vi "prototype UI_RESONANT.vi"() -> ()   [LabVIEW 2012]
uses:
  Custom Controls/Ch selector.ctl
  Custom Controls/MAIN Image panel reso tab Control type def.ctl
  Custom Controls/scan mode main settings tab.ctl
  Custom Controls/pixel resolution enum.ctl
  Custom Controls/advanced settings inner tab CTL.ctl
  Custom Controls/Histogram tab reso.ctl
  Custom Controls/file format type def.ctl
  Custom Controls/experiment type.ctl
  Custom Controls/display palette control.ctl
  <vilib>/event_ctls.llb/lveventtype.ctl
  GFG/GFG library.lvlib
panel:
  in  "reset zoom":bool
  in  "bool.stage.speed":bool
  in  "Objective":u16(ring) items=["10x Olympus", "20x Nikon", "30x Zeiss"]
  in  "x.voltage":dbl=0.9999999999999999 min=0.0 max=5.5 step=0.1
  in  "y.voltage":dbl=1.0 min=0.0 max=5.5 step=0.1
  in  "y.volt.offset":dbl=-0.2 step=0.1
  in  "x.volt.offset":dbl=-0.2 step=0.1
  in  "shutter":bool
  in  "x.pixels":i32=256 min=2 max=2048 step=2
  in  "clear prot":bool
  in  "timestamp.prot":bool
  in  "protocol.notes":string caption="notebook"
  in  "pos \nstore F":bool
  in  "pos \nstore E":bool
  in  "pos \nstore D":bool
  in  "pos \nstore C":bool
  in  "pos \nstore B":bool
  in  "pos \nstore A":bool
  out "String 10":string
  in  "pos \nrecall F":bool
  in  "pos \nrecall E":bool
  in  "pos \nrecall D":bool
  in  "pos \nrecall C":bool
  in  "pos \nrecall B":bool
  in  "pos \nrecall A":bool
  out "String 11":string
  in  "ref img\nOpen Files Button":bool
  in  "ref img\nstore F":bool
  in  "ref img\nstore E":bool
  in  "ref img\nstore D":bool
  in  "ref img\nstore C":bool
  in  "ref img\nstore B":bool
  in  "ref img\nstore A":bool
  out "String 17":string
  in  "ref img\nSave As Button":bool
  in  "Open All\nSettings":bool
  in  "step.size.z":u16(ring)=6 items=["  1"=1, "  2"=2, "  5"=5, " 10"=10, " 20"=20, " 50"=50, "100"=100]
  in  "Stage Stop":bool
  out "frame count":dbl(slide) scale=-1.0..500.0
  in  "scan mode main settings":T1
  in  "x.correction":dbl(slide)=30.0 min=-100.0 max=100.0 step=1.0 scale=-100.0..100.0 scale format="%#_3g"
  in  "Start.Delay":dbl(slide)=220.0 min=1.0 max=320.0 step=1.0 scale=1.0..320.0 scale format="%#_3g"
  in  "pixel resolution":T2
  in  "ZOOM":dbl(slide)=1.0 min=1.0 max=16.0 step=0.1 scale=1.0..16.0 scale format="%_2g"
  in  "no. of frames to acquire":i32=10000 min=2 max=2147483646 step=2
  in  "x.fov":dbl caption="Field of view    x" format="%#_3p"
  in  "y.fov":dbl caption="y" format="%#_3p"
  out "frames.p.sec":dbl caption="frames/s" format="%#.2g"
  in  "resonant.correction.enable":bool
  out "pixels per line":i32=10000 min=2 max=2147483646 step=2
  out "lines per second":i32=10000 min=2 max=2147483646 step=2
  in  "linescan.y.pixels":i32=256 caption="Lines to display at once" min=2 max=2048 step=2
  in  "no. of lines to acquire":i32=10000 min=2 max=2147483646 step=2
  in  "save.ch.1":bool caption="ch 1"
  in  "save.ch.2":bool caption="ch 2"
  in  "save.ch.3":bool caption="ch 3"
  in  "save.ch.4":bool caption="ch 4"
  in  "save.ch.5":bool caption="ch 5"
  in  "experiment type":T3
  in  "experiment name":string
  in  "root.path":path=path "g:/"
  in  "file format":T4
  out "stack.duration":i32=10 caption="stack.duration (sec)" min=0 max=2147483646 step=2
  in  "add":bool
  in  "clear all":bool
  in  "clear last":bool
  in  "move to z.stack.\nstart plane":bool
  in  "start z.stack":bool
  in  "frames.per.plane":i32=10000
  in  "z.spacing":dbl=1.0 caption="z.spacing (um)" min=0.1 step=0.1
  out "no of planes":i32=10 min=0 max=2147483646 step=2
  in  "piezo.mode":bool
  in  "frames.per.z.cycle":dbl=2.0 min=3.0 max=101.0 step=2.0
  in  "piezo.active":bool
  in  "Z UP":bool
  in  "Z DOWN":bool
  out "String 7":string
  in  "step.size.xy":u16(ring)=6 items=["  1"=1, "  2"=2, "  5"=5, " 10"=10, " 20"=20, " 50"=50, "100"=100]
  in  "Y UP":bool
  in  "X LEFT":bool
  in  "Y DOWN":bool
  in  "X RIGHT":bool
  out "String 6":string
  in  "setY":dbl caption="Z-Stepper" format="%#.1f"
  in  "setX":dbl caption="Z-Stepper" format="%#.1f"
  in  "setZ":dbl caption="set" format="%#.1f"
  out "String 4":string
  out "posZ":dbl caption="actual" format="%#.1f"
  out "posX":dbl caption="Z-Stepper" format="%#.1f"
  out "posY":dbl caption="Z-Stepper" format="%#.1f"
  out "String 3":string
  in  "QUIT":bool
  in  "Record":bool
  in  "FOCUS":bool
  in  "MAIN Image panels reso":T5
  out "Channel 1 large":T6(plugin-control)
  out "Channel 2 large":T6(plugin-control)
  out "Channel 3 large":T6(plugin-control)
  out "Channel 4 large":T6(plugin-control)
  out "Channel 5 large":T6(plugin-control)
  out "Channel 1 small":T6(plugin-control)
  out "Channel 2 small":T6(plugin-control)
  out "Channel 4 small":T6(plugin-control)
  out "Channel 3 small":T6(plugin-control)
  in  "Blue Channel (Overlay)":T7 caption="B"
  in  "Green Channel (Overlay)":T7=enum."Ch 1" caption="G"
  in  "Red Channel (Overlay)":T7=enum."Ch 2" caption="R"
  out "RGB overlay":T6(plugin-control)
  out "ROI chart":sgl[][](graph)=[[54.570076, 54.556858]]
  in  "ROI channel":T7=enum."Ch 1" caption="Channel"
  out "ROI Image display":T6(plugin-control)
  in  "confirm line":bool
  in  "channel arb line scan":T7 caption="Channel"
  out "arb line scan display":T6(plugin-control)
  in  "Cancel":bool
  in  "hist/ref slider tab":enum32{" "}(tab)
  in  "display every n-th frame":i8=4 min=2 step=1
  in  "PIN Button hist/ref slider tab":bool
  in  "Histograms tab reso":T8
  in  "auto scale\n      CH 1":bool=TRUE caption="auto scale 2"
  in  "Min Max Channel 1":cluster{dbl, dbl}(slide) scale=-32768.0..32767.0 scale format="%#_5g"
  out "Histogram 1":T9(graph)
  out "String 12":string
  in  "auto scale\n      CH 4":bool=TRUE caption="auto scale 2"
  in  "Min Max Channel 4":cluster{dbl, dbl}(slide) scale=-100.0..2047.0 scale format="%#_4g"
  out "Histogram 4":T9(graph)
  out "String 15":string
  in  "auto scale\n      CH 5":bool=TRUE caption="auto scale 2"
  in  "Min Max Channel 5":cluster{dbl, dbl}(slide) scale=-100.0..2047.0 scale format="%#_4g"
  out "Histogram 5":T9(graph)
  out "String 16":string
  in  "auto scale\n      CH 3":bool=TRUE caption="auto scale 2"
  in  "Min Max Channel 3":cluster{dbl, dbl}(slide) scale=-32768.0..32767.0 scale format="%#.1f"
  out "Histogram 3":T9(graph)
  out "String 14":string
  in  "auto scale\n      CH 2":bool=TRUE caption="auto scale 2"
  in  "Min Max Channel 2":cluster{dbl, dbl}(slide) scale=-32768.0..32767.0 scale format="%#.0f"
  out "Histogram 2":T9(graph)
  out "String 13":string
  in  "avg type":u16(ring) items=["none", "group avg", "moving avg"]
  in  "avg of":i8=10 min=2 step=1
  in  "display palette":T10
  in  "laser power slider tab":enum32{""}(tab)
  in  "enable set power max":bool
  in  "set power max":bool
  in  "Laser Power":dbl(knob) min=0.0 max=100.0 step=0.5 scale=0.0..100.0 scale format="%3d"
  in  "PIN Button laser power slider tab":bool
  in  "PMT slider tab":enum32{""}(tab)
  in  "PMT 2":u16(slide) max=1000 scale=0.0..1000.0
  in  "PMT 1":u16(slide) max=1250 scale=0.0..1000.0
  out "String 5":string
  in  "PMT 4":u16(slide) max=1000 scale=0.0..1000.0
  in  "PMT 3":u16(slide) max=1250 scale=0.0..1000.0
  out "String 18":string
  in  "PIN Button PMT slider tab":bool
  in  "advanced settings slider tab":enum32{""}(tab)
  in  "advanced settings inner tab":T11
  in  "y.pixel.sz":dbl=1e-05 min=1e-09 max=1e-05 step=1e-07 format="%#_3p"
  in  "x.pixel.sz":dbl=1e-05 min=1e-09 max=1e-05 step=1e-07 format="%#_3p"
  in  "y.pixels":i32=256 caption="Y Resolution" min=2 max=2048 step=2
  in  "nomin.x.pixels":i32=256 caption="X resolution" min=2 max=2048 step=2
  in  "voltage.for\nmin.field.of.view\nresonant":dbl=5.0
  in  "max.field.of.view\nresonant":dbl=300.0 format="%#_6p"
  in  "voltage.for\nmax.field.of.view\nresonant":dbl=5.0
  in  "max.field.of.view":dbl=300.0 format="%#_6p"
  in  "voltage.for\nmax.field.of.view":dbl=5.0
  in  "external.start.trigger.enable":bool=TRUE caption="WAIT FOR TRIGGER"
  in  "pos  pockels cell PMT Data":dbl[][](array[numeric])=[[0.0, 0.0], [1.0, 0.0]] caption="Data" format="%0.1f"
  out "interpol XY":cluster{dbl[], "Best Exponential Fit":dbl[]}[](graph)
  in  "PIN Button advanced settings slider tab":bool
  in  "XYZ stage settings slider tab":enum32{" "}(tab)
  in  "set stage speed":bool
  in  "enable virtual XYZ":bool
  out "String 19":string
  in  "set Y to zero":bool
  in  "set X to zero":bool
  in  "set all to zero":bool
  in  "set Z to zero":bool
  out "String 9":string
  in  "reverse y":bool
  in  "reverse x":bool
  in  "reverse z":bool
  out "String 8":string
  in  "PIN Button XYZ stage settings slider tab":bool
  in  "SCIENTIFICA Button":bool
  # "to zoom out press and hold Shift"
  # "current pos."
  # "go to pos."
  # "STORE positions"
  # "RECALL  positions"
  # "REFERENCE IMAGES"
  # "STORE"
  # "CHANNELS TO SAVE"
  # "zig-zag (leaf scan)"
  # "planes"
  # "1"
  # "2"
  # "3"
  # "4"
  # "Press and hold Ctrl to add multiple ROIs"
  # "This checkbox is only for starting the image acquisition using a TTL rising edge trigger from an external device. Don't tick this box unless an incoming trigger is wired up, otherwise the software may freeze. To reset, click QUIT and restart. If you want to send a trigger to an external device, just connect the ai.start.trigger.channel (e.g.PFI2, specified in settings.INI) to the external device, but leave the  checkbox above unticked."
  # "Z"
  # "laser"
  # "virtual XYZ"
  # "set zero"
  # "reverse \ndirection"
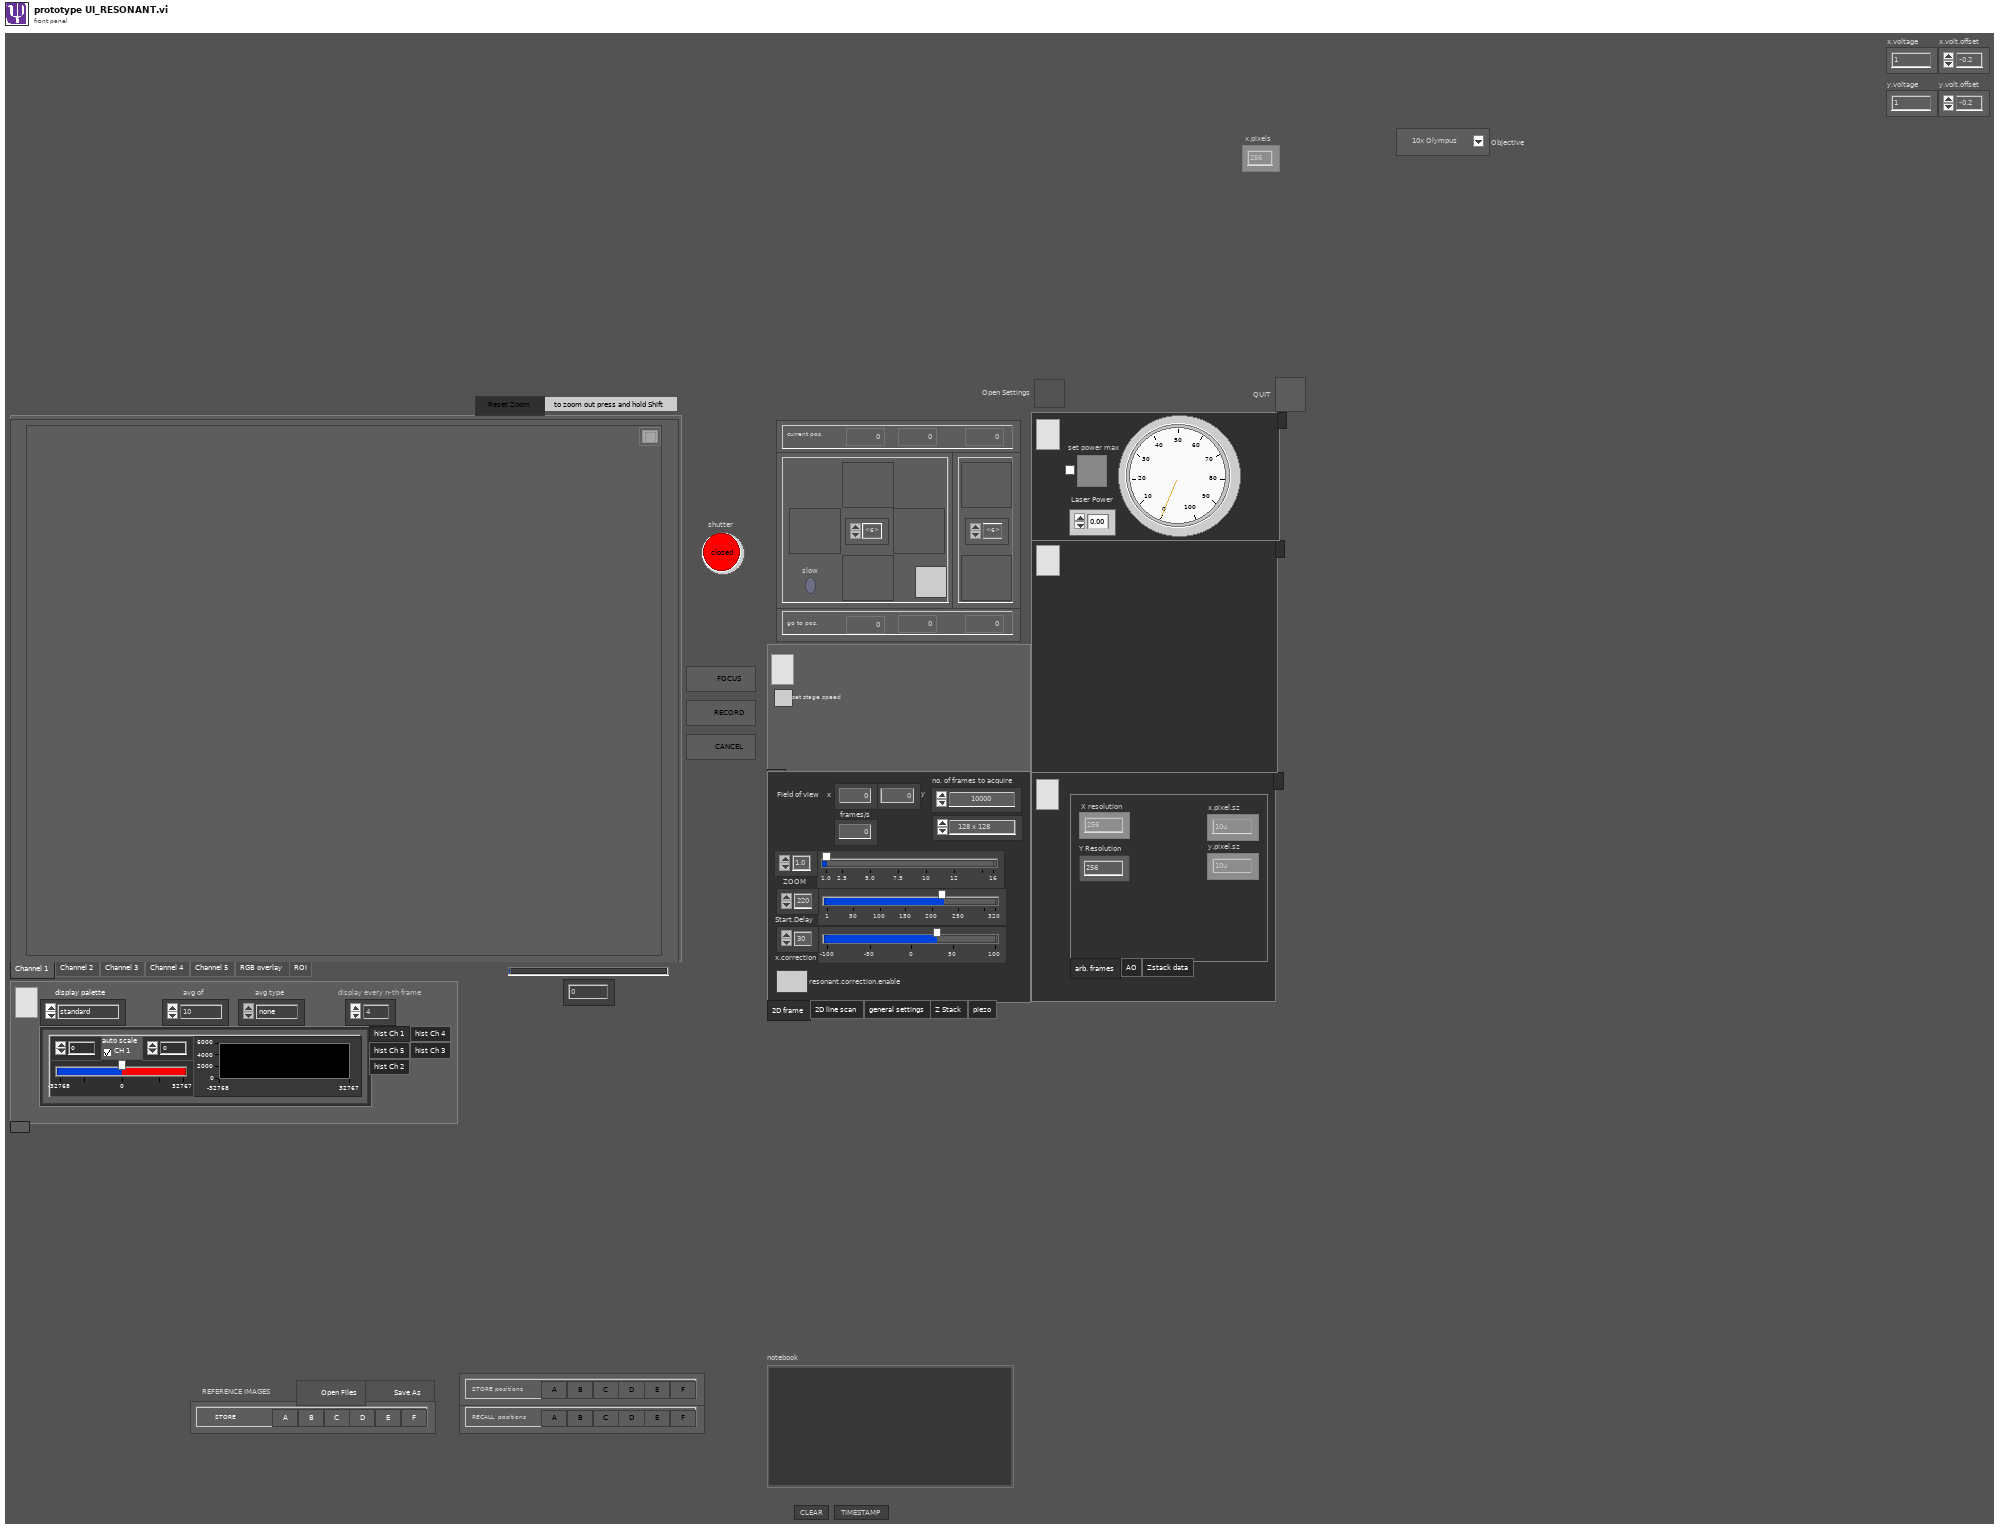
[diagram p1: front panel]
types:
  T1 = typedef "scan mode main settings tab.ctl" = enum32{"2D frame", "2D line scan", "general settings", "Z Stack", "piezo"}
  T2 = typedef "pixel resolution enum.ctl" = enum16{"   128 x 128", "   256 x 128", "   256 x 256", "   512 x  64", "   512 x 128", "   512 x 256", "   512 x 512", "  1024 x 512", "  1024 x 1024", "   arbitrary"}
  T3 = typedef "experiment type.ctl" = string
  T4 = typedef "file format type def.ctl" = enum16{"16bit raw", "32bit raw", "16bit multi-tiff (interleave)", "16bit multi-tiff (separate)", "16bit multi-tiff (stacked)", "32bit multi-tiff (interleave)", "32bit multi-tiff (separate)", "32bit multi-tiff (stacked)", "16bit tiff series (interleave)", "16bit tiff series (separate)", "16bit tiff series (stacked)", "32bit tiff series (interleave)", "32bit tiff series (separate)", "32bit tiff series (stacked)"}
  T5 = typedef "MAIN Image panel reso tab Control type def.ctl" = enum32{"Channel 1", "Channel 2", "Channel 3", "Channel 4", "Channel 5", "all channels", "RGB overlay", "ROI", "arbitrary line scan"}
  T6 = typedef "IMAQ Image.ctl" = refnum<image>
  T7 = typedef "Ch selector.ctl" = enum16{"none", "Ch 1", "Ch 2", "Ch 3", "Ch 4", "Ch 5"}
  T8 = typedef "Histogram tab reso.ctl" = enum32{"hist Ch 1", "hist Ch 4", "hist Ch 5", "hist Ch 3", "hist Ch 2"}
  T9 = cluster{"Starting Value":sgl, "Incremental Value":sgl, "Histogram":u32[]}
  T10 = typedef "display palette control.ctl" = enum16{"standard", "high clipping red", "low clipping blue", "high and low clipping"}
  T11 = typedef "advanced settings inner tab CTL.ctl" = enum32{"arb. frames", "AO", "AI", "channels", "trigger", "Zstack data"}
  T12 = enum8{"Enabled", "Disabled", "Disabled and Grayed Out"}
  T13 = typedef "Image Type" = u32
  T14 = cluster{refnum<vi>, refnum<vi>, refnum<vi>, refnum<vi>, refnum<vi>, refnum<vi>, refnum<vi>, refnum<vi>, refnum<vi>, refnum<vi>, refnum<vi>, refnum<vi>}
  T15 = cluster{"New Image":T6, "New Image":T6, "New Image":T6, "New Image":T6, "New Image":T6, "New Image":T6, "New Image":T6, "New Image":T6, "New Image":T6, "New Image":T6, "New Image":T6, "New Image":T6}
  T16 = typedef "lveventtype.ctl" = enum32{"Null", "Timeout", "Annotation Menu Selection", "Annotation Menu Selection?", "App Instance Close", "App Instance Close?", "Autoscale Range Change", "Cell Edit", "Cell Edit?", "Cursor Grab", "Cursor Grab?", "Cursor Menu Selection", "Cursor Menu Selection?", "Cursor Move", "Cursor Release", "Data Change", "Direction Change", "Display State Change", "Drag Ended", "Drag Enter", "Drag Leave", "Drag Over", "Drag Source Update", "Drag Starting", "Drag Starting?", "Drop", "Exec State Change", "Key Down", "Key Down?", "Key Repeat", "Key Repeat?", "Key Up", "Listbox Double Click", "Menu Activation?", "Menu Selection (App)", "Menu Selection? (App)", "Menu Selection (User)", "Mouse Down", "Mouse Down?", "Mouse Enter", "Mouse Leave", "Mouse Move", "Mouse Up", "NI Security User Change (App)", "Pane Size", "Panel Close", "Panel Close?", "Panel Resize", "Plot Attribute Change", "Scale Range Change", "Shortcut Menu Activation?", "Shortcut Menu Selection (App)", "Shortcut Menu Selection? (App)", "Shortcut Menu Selection (User)", "Tree Double Click", "Tree Drag", "Tree Drag?", "Tree Drop", "Tree Drop?", "Tree Item Close", "Tree Item Close?", "Tree Item Open", "Tree Item Open?", "Value Change"}
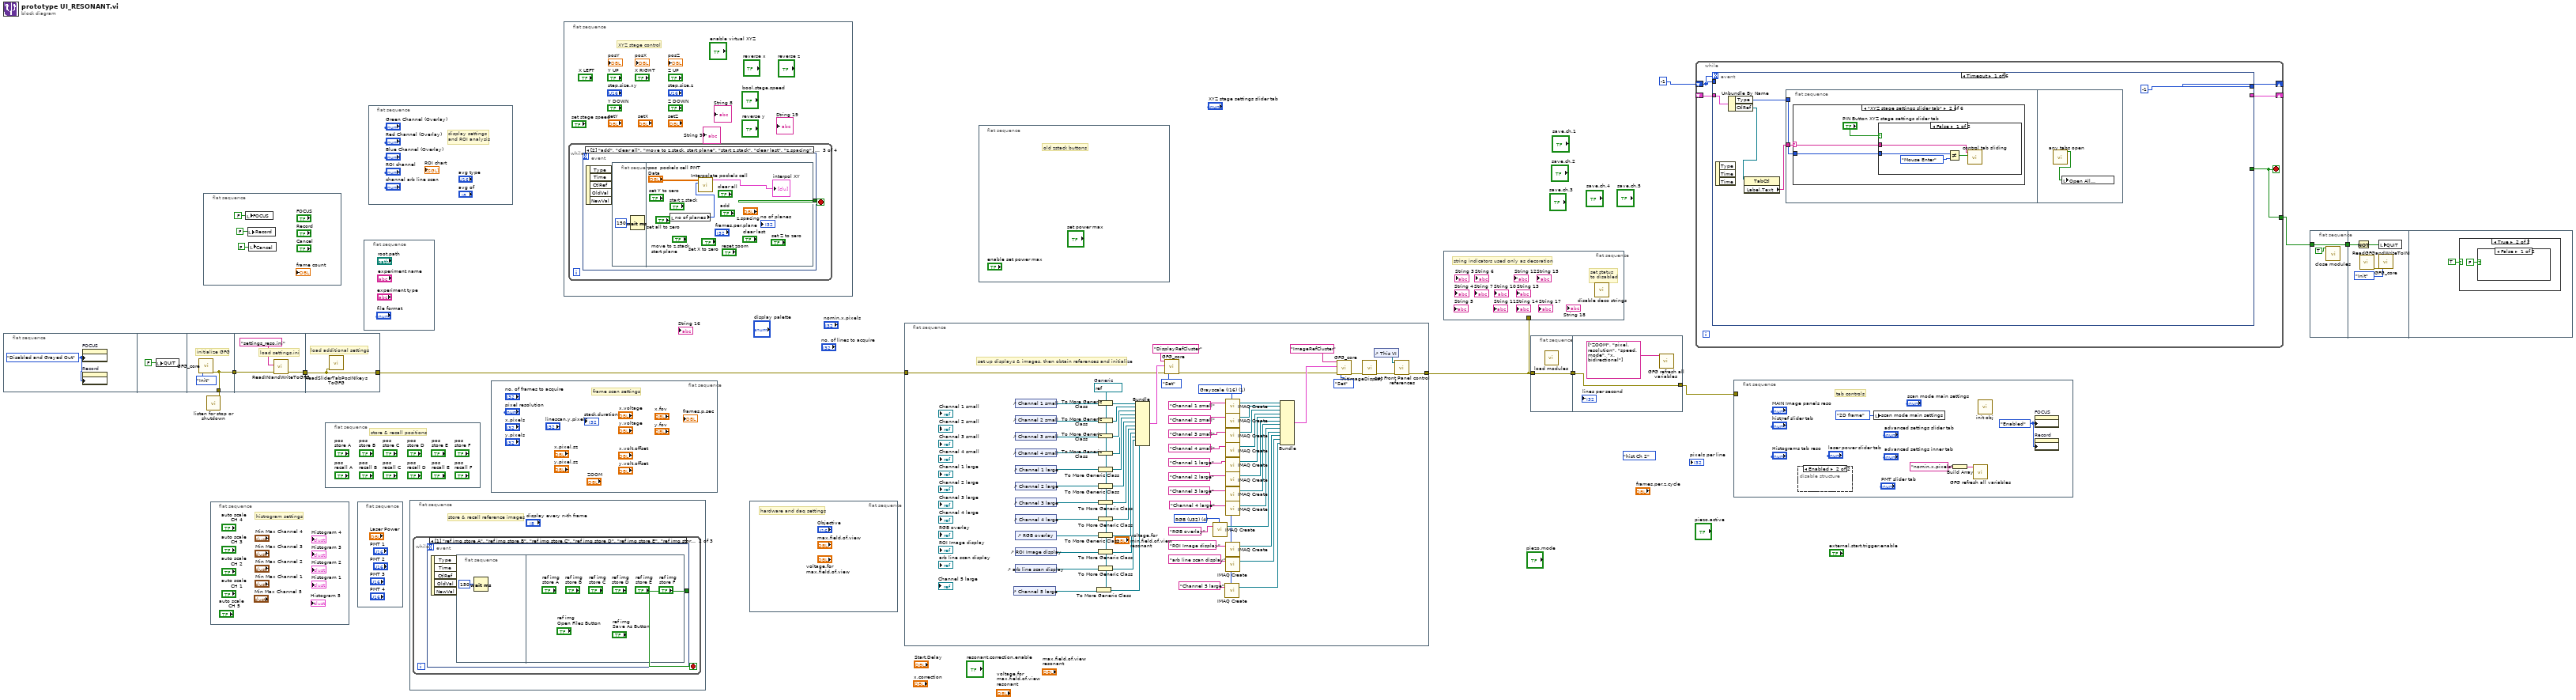
[diagram p0: block diagram]
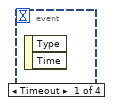
[diagram p2: hidden frame]
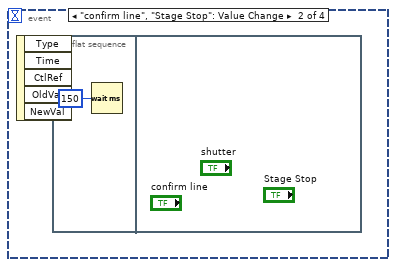
[diagram p3: hidden frame]
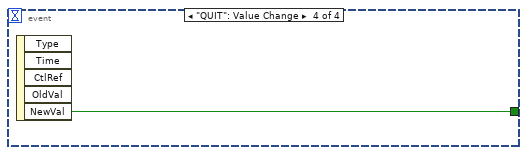
[diagram p4: hidden frame]
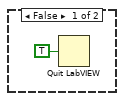
[diagram p5: hidden frame]
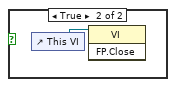
[diagram p6: hidden frame]
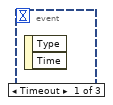
[diagram p7: hidden frame]
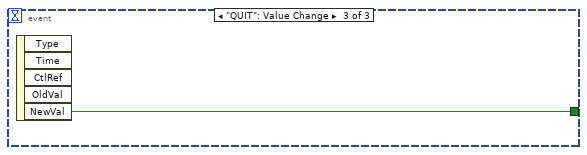
[diagram p8: hidden frame]
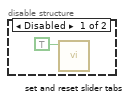
[diagram p9: hidden frame]
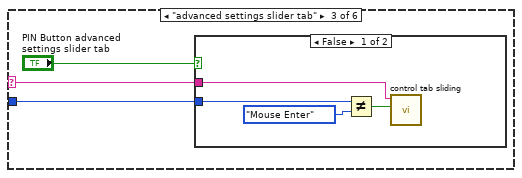
[diagram p12: hidden frame]
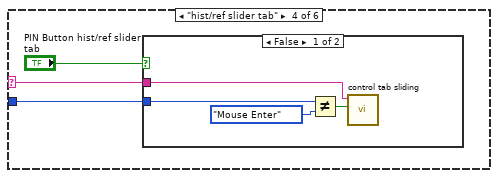
[diagram p14: hidden frame]
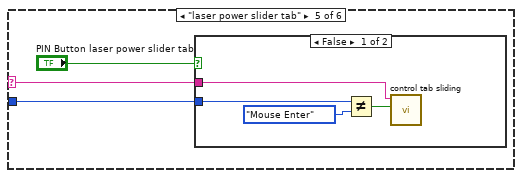
[diagram p16: hidden frame]
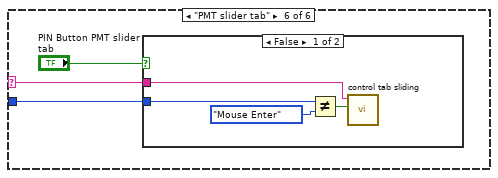
[diagram p18: hidden frame]
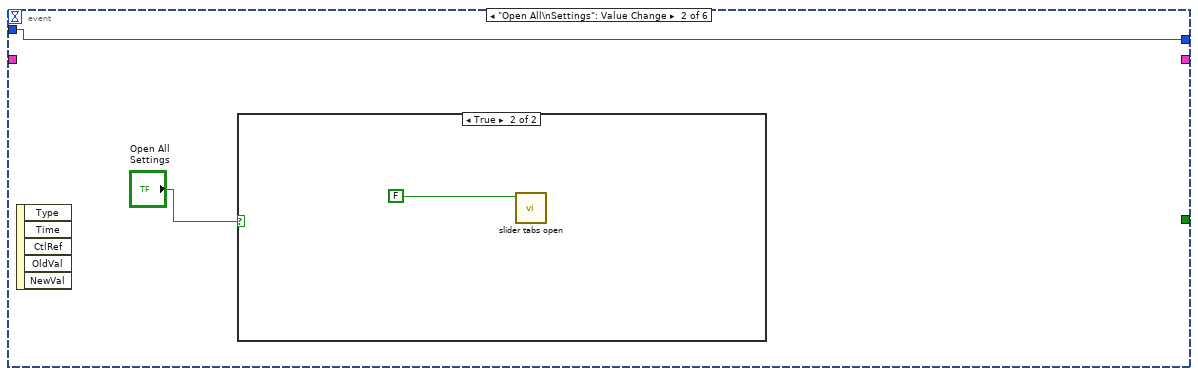
[diagram p20: hidden frame]
diagram:
  (unwired) Histogram_tab_reso."hist Ch 2" ("Histograms tab reso")
  n1 = flat-sequence {
    tunnel: [w13] -> w10
    tunnel: [w13] -> w9
    tunnel: w10 -> [w17]
    tunnel: [w16] -> w3
    tunnel: [w18] -> w6
    tunnel: w3 -> [w18]
    frame #0 {
      w11 = T12."Disabled and Grayed Out" ("Disabled")
      n2 = property on="FOCUS" class="Bool (strict)"("DisabledEnum"=w11) -> ()  [unwired: 2 in, 2 out]
      n3 = property on="Record" class="Bool (strict)"("DisabledEnum"=w11) -> ()  [unwired: 2 in, 2 out]
    }
    frame #1 {
      n4 = local write "QUIT"(FALSE ("QUIT")) -> ()
    }
    frame #2 {
      # "initialize GFG"
      n5 = call "GFG_core.vi"("Action"=enum16{"Init", "Set", "Get"}."Init") -> ("error out"=w13:errorcluster)  [unwired: 12 in, 6 out]
    }
    frame #3 {
      # "load settings.ini"
      n6 = call "ReadINIandWriteToGFG.vi"("error in (no error)"=w17, "name or relative path"="settings_reso.ini") -> ("error out"=w16:errorcluster)  [unwired: 9 in]
    }
    frame #4 {
      # "load additional settings"
      n7 = call "ReadSliderTabPosINIkeysToGFG.vi"("error in (no error)"=w18) -> ()  [unwired: 11 in]
    }
  }
  n8 = flat-sequence {
    frame #0 {
      n9 = local write "FOCUS"(FALSE ("FOCUS")) -> ()
      n10 = local write "Record"(FALSE ("Record")) -> ()
      n11 = local write "Cancel"(FALSE ("Cancel")) -> ()
    }
  }
  n12 = call "listen for stop or shutdown.vi"("error in (no error)"=w9) -> ()  [unwired: 9 in, 2 out]
  n13 = flat-sequence {
    frame #0 {
      # "histrogram settings"
    }
  }
  n14 = flat-sequence {
    frame #0 {
      # "store & recall positions"
    }
  }
  n15 = flat-sequence {
    frame #0 {
    }
  }
  n16 = flat-sequence {
    frame #0 {
    }
  }
  n17 = flat-sequence {
    frame #0 {
      # "display settings\nand ROI analysis"
    }
  }
  n18 = flat-sequence {
    frame #0 {
      # "store & recall reference images"
      n19 = while {
        stop <- w22 stop-if-true
        n20 = event shown="[1] \"ref img store A\", \"ref img store B\", \"ref img store C\", \"ref img store D\", \"ref img store E\", \"ref img store F\", \"ref img Save As Button\", \"ref img Open Files Button\": Value Change" {
          selector: _ -> [_ _ _]
          dyn-events: _ -> [_ _ _]
          timeout: _ -> [_ _ _]
          tunnel: [_ _ w24] -> w22
          event Timeout {
            n21 = event-data() -> ()  [unwired: 1 in, 2 out]
          }
          event "ref img\nstore A", "ref img\nstore B", "ref img\nstore C", "ref img\nstore D", "ref img\nstore E", "ref img\nstore F", "ref img\nSave As Button", "ref img\nOpen Files Button": Value Change {
            n22 = event-data() -> ()  [unwired: 1 in, 5 out]
            n23 = flat-sequence {
              frame #0 {
                n24 = Wait (ms)(milliseconds to wait=u32 150) -> ()  [unwired: 1 out]
              }
              frame #1 {
              }
            }
          }
          event "QUIT": Value Change {
            n25 = event-data() -> ("NewVal"=w24:bool)  [unwired: 1 in, 4 out]
          }
        }
      }
    }
  }
  n26 = flat-sequence {
    frame #0 {
      # "frame scan settings"
    }
  }
  n27 = flat-sequence {
    frame #0 {
      # "XYZ stage control"
      n28 = while {
        stop <- w25 stop-if-true
        n29 = event shown="[2] \"add\", \"clear all\", \"move to z.stack. start plane\", \"start z.stack\", \"clear last\", \"z.spacing\", \"frames.per.plane\", \"no of planes\", \"set Y to zero\", \"set X to zero\", \"set all to zero\", \"set Z to zero\", \"reset zoom\": Value Change" {
          selector: _ -> [_ _ _ _]
          dyn-events: _ -> [_ _ _ _]
          timeout: _ -> [_ _ _ _]
          tunnel: [_ _ _ w31] -> w25
          event Timeout {
            n30 = event-data() -> ()  [unwired: 1 in, 2 out]
          }
          event "confirm line", "Stage Stop": Value Change {
            n31 = event-data() -> ()  [unwired: 1 in, 5 out]
            n32 = flat-sequence {
              frame #0 {
                n33 = Wait (ms)(milliseconds to wait=u32 150) -> ()  [unwired: 1 out]
              }
              frame #1 {
              }
            }
          }
          event "add", "clear all", "move to z.stack.\nstart plane", "start z.stack", "clear last", "z.spacing", "frames.per.plane", "no of planes", "set Y to zero", "set X to zero", "set all to zero", "set Z to zero", "reset zoom": Value Change {
            n34 = event-data() -> ()  [unwired: 1 in, 5 out]
            n35 = flat-sequence {
              frame #0 {
                n36 = Wait (ms)(milliseconds to wait=u32 150) -> ()  [unwired: 1 out]
              }
              frame #1 {
                n37 = local read "no of planes"() -> (w30:i32)
                n38 = call "Interpolate pockels cell.vi"("nr of planes"=w30, "Data"="pos  pockels cell PMT Data") -> ("Raw Data and Interpolated Data"=→"interpol XY":cluster{dbl[], "Best Exponential Fit":dbl[]}[])  [unwired: 8 in, 1 out]
              }
            }
          }
          event "QUIT": Value Change {
            n39 = event-data() -> ("NewVal"=w31:bool)  [unwired: 1 in, 4 out]
          }
        }
      }
    }
  }
  n40 = flat-sequence {
    frame #0 {
      # "hardware and daq settings"
    }
  }
  n41 = flat-sequence {
    tunnel: [w51] -> w7
    tunnel: w6 -> [w50]
    frame #0 {
      w38 = T13 4 items=["Grayscale (U8)", "Grayscale (I16)", "Grayscale (SGL)", "Complex (CSG)", "RGB (U32)", "HSL (U32)", "RGB (U64)", "Grayscale (U16)"] ("Image Type")
      w33 = T13 1 items=["Grayscale (U8)", "Grayscale (I16)", "Grayscale (SGL)", "Complex (CSG)", "RGB (U32)", "HSL (U32)", "RGB (U64)", "Grayscale (U16)"] ("Image Type")
      w36 = refnum<vi> refnum  # Generic
      # "set up displays & images, then obtain references and initialize"
      n42 = control-ref of="Channel 5 large"() -> (w37:refnum<vi>)
      n43 = control-ref of="Channel 1 small"() -> (w49:refnum<vi>)
      n44 = control-ref of="Channel 2 small"() -> (w48:refnum<vi>)
      n45 = control-ref of="Channel 3 small"() -> (w47:refnum<vi>)
      n46 = control-ref of="Channel 4 small"() -> (w46:refnum<vi>)
      n47 = control-ref of="Channel 1 large"() -> (w45:refnum<vi>)
      n48 = control-ref of="Channel 2 large"() -> (w44:refnum<vi>)
      n49 = control-ref of="Channel 3 large"() -> (w43:refnum<vi>)
      n50 = control-ref of="Channel 4 large"() -> (w42:refnum<vi>)
      n51 = control-ref of="RGB overlay"() -> (w41:refnum<vi>)
      n52 = control-ref of="ROI Image display"() -> (w40:refnum<vi>)
      n53 = control-ref of="arb line scan display"() -> (w39:refnum<vi>)
      n54 = To More Generic Class(target class=w36, reference=w37) -> (generic class reference=w35:refnum<vi>)
      n55 = To More Generic Class(target class=w36, reference=w49) -> (generic class reference=w91:refnum<vi>)
      n56 = To More Generic Class(target class=w36, reference=w48) -> (generic class reference=w84:refnum<vi>)
      n57 = To More Generic Class(target class=w36, reference=w47) -> (generic class reference=w83:refnum<vi>)
      n58 = To More Generic Class(target class=w36, reference=w46) -> (generic class reference=w82:refnum<vi>)
      n59 = To More Generic Class(target class=w36, reference=w45) -> (generic class reference=w81:refnum<vi>)
      n60 = To More Generic Class(target class=w36, reference=w44) -> (generic class reference=w90:refnum<vi>)
      n61 = To More Generic Class(target class=w36, reference=w43) -> (generic class reference=w89:refnum<vi>)
      n62 = To More Generic Class(target class=w36, reference=w42) -> (generic class reference=w88:refnum<vi>)
      n63 = To More Generic Class(target class=w36, reference=w41) -> (generic class reference=w87:refnum<vi>)
      n64 = To More Generic Class(target class=w36, reference=w40) -> (generic class reference=w86:refnum<vi>)
      n65 = To More Generic Class(target class=w36, reference=w39) -> (generic class reference=w85:refnum<vi>)
      n66 = Bundle(w91, w84, w83, w82, w81, w90, w89, w88, w87, w86, w85, w35) -> (w94:T14)  [unwired: 1 in]
      n67 = call "GFG_core.vi"("Variable Name in"="DisplayRefCluster", "Variant in"=w94, "error in (no error)"=w50, "Action"=enum16{"Init", "Set", "Get"}."Set") -> ("error out"=w55:errorcluster)  [unwired: 9 in, 6 out]
      n68 = call "IMAQ Create"("Image Name"="RGB overlay", "Image Type"=w38) -> ("New Image"=w75:T6)  [unwired: 3 in, 1 out]
      n69 = call "IMAQ Create"("Image Name"="Channel 5 large", "Image Type"=w33) -> ("New Image"=w32:T6)  [unwired: 3 in, 1 out]
      n70 = call "IMAQ Create"("Image Name"="Channel 1 small", "Image Type"=w33) -> ("New Image"=w67:T6)  [unwired: 3 in, 1 out]
      n71 = call "IMAQ Create"("Image Name"="Channel 2 small", "Image Type"=w33) -> ("New Image"=w68:T6)  [unwired: 3 in, 1 out]
      n72 = call "IMAQ Create"("Image Name"="Channel 3 small", "Image Type"=w33) -> ("New Image"=w69:T6)  [unwired: 3 in, 1 out]
      n73 = call "IMAQ Create"("Image Name"="Channel 4 small", "Image Type"=w33) -> ("New Image"=w70:T6)  [unwired: 3 in, 1 out]
      n74 = call "IMAQ Create"("Image Name"="Channel 1 large", "Image Type"=w33) -> ("New Image"=w71:T6)  [unwired: 3 in, 1 out]
      n75 = call "IMAQ Create"("Image Name"="Channel 2 large", "Image Type"=w33) -> ("New Image"=w72:T6)  [unwired: 3 in, 1 out]
      n76 = call "IMAQ Create"("Image Name"="Channel 3 large", "Image Type"=w33) -> ("New Image"=w73:T6)  [unwired: 3 in, 1 out]
      n77 = call "IMAQ Create"("Image Name"="Channel 4 large", "Image Type"=w33) -> ("New Image"=w74:T6)  [unwired: 3 in, 1 out]
      n78 = call "IMAQ Create"("Image Name"="ROI Image display", "Image Type"=w33) -> ("New Image"=w76:T6)  [unwired: 3 in, 1 out]
      n79 = call "IMAQ Create"("Image Name"="arb line scan display", "Image Type"=w33) -> ("New Image"=w77:T6)  [unwired: 3 in, 1 out]
      n80 = Bundle("New Image"=w67, "New Image"=w68, "New Image"=w69, "New Image"=w70, "New Image"=w71, "New Image"=w72, "New Image"=w73, "New Image"=w74, "New Image"=w75, "New Image"=w76, "New Image"=w77, "New Image"=w32) -> (w79:T15)  [unwired: 1 in]
      n81 = call "GFG_core.vi"("Variable Name in"="ImageRefCluster", "Variant in"=w79, "error in (no error)"=w55, "Action"=enum16{"Init", "Set", "Get"}."Set") -> ("error out"=w54:errorcluster)  [unwired: 9 in, 6 out]
      n82 = call "InitImageDisplay.vi"("error in (no error)"=w54) -> ("error out"=w53:errorcluster)  [unwired: 10 in]
      n83 = control-ref of="This VI"() -> (w52:refnum<vi>)
      n84 = call "get Front Panel control references.vi"("error in (no error)"=w53, "Main VI"=w52) -> ("error out"=w51:errorcluster)  [unwired: 9 in]
    }
  }
  n85 = flat-sequence {
    frame #0 {
      # "old zstack buttons"
    }
  }
  n86 = flat-sequence {
    tunnel: w7 -> [_]
    frame #0 {
      # "set status\nto disabled"
      # "string indicators used only as decoration"
      n87 = call "disable deco strings.vi"() -> ()  [unwired: 11 in, 1 out]
    }
  }
  n88 = flat-sequence {
    tunnel: w7 -> [w95]
    tunnel: [w95] -> w2
    tunnel: [w97] -> w1
    tunnel: w2 -> [w97]
    frame #0 {
      n89 = call "load modules.vi"() -> ()  [unwired: 12 in]
    }
    frame #1 {
      n90 = call "GFG refresh all variables.vi"("All Variable Names"=string[] ["ZOOM", "pixel.resolution", "speed.mode", "x.bidirectional"] ("Variables Names In")) -> ()  [unwired: 11 in]
    }
  }
  n91 = while {
    tunnel: [w102] -> w8
    shift-right: [w101] -> _
    shift-left: _ -> [w99]
    shift-right: [w100] -> _
    shift-left: -1 -> [w98]
    stop <- w102 stop-if-true
    n92 = event shown="[0] Timeout" {
      selector: _ -> [_ _ _ _ _ _]
      dyn-events: _ -> [_ _ _ _ _ _]
      timeout: w98 -> [_ _ _ _ _ _]
      tunnel: [_ _ "QUIT" _ _ _] -> w102
      tunnel: [_ _ _ _ w162 _] -> w101
      tunnel: [-1 w146 w157 w159 w166 w176] -> w100
      tunnel: w99 -> [w107 _ _ _ w161 _]
      tunnel: w98 -> [_ w146 w157 w159 w165 w176]
      event Timeout {
        n93 = event-data() -> ()  [unwired: 1 in, 3 out]
        n94 = Unbundle By Name(w107) -> ("Type"=w104:T16, "CtlRef"=w106:refnum<vi>)
        n95 = property class="TabCtl"(reference=w106) -> ("Label.Text"=w105:string)  [unwired: 1 in, 2 out]
        n96 = flat-sequence {
          tunnel: w105 -> [w109]
          tunnel: w104 -> [w108]
          frame #0 {
            n97 = case shown="\"XYZ stage settings slider tab\"" w109 {
              selector: w109 -> [_ w112 w117 w126 w131 w140]
              tunnel: w108 -> [_ w111 w118 w124 w132 w139]
              frame "False", Default {
              }
              frame "XYZ stage settings slider tab" {
                n98 = case shown="False" "PIN Button XYZ stage settings slider tab" {
                  tunnel: w112 -> [w116 _]
                  tunnel: w111 -> [w115 _]
                  frame False {
                    n99 = Not Equal?(x=w115, y=lveventtype."Mouse Enter" ("Type")) -> (x != y?=w114:bool)
                    n100 = call "control tab sliding.vi"("close(T)/open(F)"=w114, "String"=w116) -> ()  [unwired: 10 in]
                  }
                  frame True {
                  }
                }
              }
              frame "advanced settings slider tab" {
                n101 = case shown="False" "PIN Button advanced settings slider tab" {
                  tunnel: w117 -> [w123 _]
                  tunnel: w118 -> [w122 _]
                  frame False {
                    n102 = Not Equal?(x=w122, y=lveventtype."Mouse Enter" ("Type")) -> (x != y?=w121:bool)
                    n103 = call "control tab sliding.vi"("close(T)/open(F)"=w121, "String"=w123) -> ()  [unwired: 10 in]
                  }
                  frame True {
                  }
                }
              }
              frame "hist/ref slider tab" {
                n104 = case shown="False" "PIN Button hist/ref slider tab" {
                  tunnel: w126 -> [w130 _]
                  tunnel: w124 -> [w129 _]
                  frame False {
                    n105 = Not Equal?(x=w129, y=lveventtype."Mouse Enter" ("Type")) -> (x != y?=w128:bool)
                    n106 = call "control tab sliding.vi"("close(T)/open(F)"=w128, "String"=w130) -> ()  [unwired: 10 in]
                  }
                  frame True {
                  }
                }
              }
              frame "laser power slider tab" {
                n107 = case shown="False" "PIN Button laser power slider tab" {
                  tunnel: w131 -> [w137 _]
                  tunnel: w132 -> [w136 _]
                  frame False {
                    n108 = Not Equal?(x=w136, y=lveventtype."Mouse Enter" ("Type")) -> (x != y?=w135:bool)
                    n109 = call "control tab sliding.vi"("close(T)/open(F)"=w135, "String"=w137) -> ()  [unwired: 10 in]
                  }
                  frame True {
                  }
                }
              }
              frame "PMT slider tab" {
                n110 = case shown="False" "PIN Button PMT slider tab" {
                  tunnel: w140 -> [w144 _]
                  tunnel: w139 -> [w143 _]
                  frame False {
                    n111 = Not Equal?(x=w143, y=lveventtype."Mouse Enter" ("Type")) -> (x != y?=w142:bool)
                    n112 = call "control tab sliding.vi"("close(T)/open(F)"=w142, "String"=w144) -> ()  [unwired: 10 in]
                  }
                  frame True {
                  }
                }
              }
            }
          }
          frame #1 {
            n113 = call "any tabs open.vi"() -> ("any tabs open?"=w145:bool)  [unwired: 11 in]
            n114 = local write "Open All\nSettings"(w145) -> ()
          }
        }
      }
      event "Open All\nSettings": Value Change {
        n115 = event-data() -> ()  [unwired: 1 in, 5 out]
        n116 = case shown="True" "Open All\nSettings" {
          frame False {
            n117 = call "slider tabs open.vi"("close(T)/open(F)"=TRUE) -> ()  [unwired: 11 in]
          }
          frame True {
            n118 = call "slider tabs open.vi"("close(T)/open(F)"=FALSE) -> ()  [unwired: 11 in]
          }
        }
      }
      event "QUIT": Value Change {
        n119 = event-data() -> ()  [unwired: 1 in, 5 out]
        n120 = call "getVIname.vi"() -> ("VI name"=w156:string)  [unwired: 19 in]
        n121 = call "SendShutdownCommand.vi"("Source VI"=w156) -> ()  [unwired: 11 in]
        n122 = call "GFG_core.vi"("Variable Name in"="shutter", "Variant in"=FALSE ("QUIT"), "Action"=enum16{"Init", "Set", "Get"}."Set") -> ()  [unwired: 10 in, 7 out]
        n123 = call "GFG_core.vi"("Variable Name in"="Cancel", "Variant in"=FALSE ("QUIT"), "Action"=enum16{"Init", "Set", "Get"}."Set") -> ()  [unwired: 10 in, 7 out]
      }
      event "SCIENTIFICA Button": Value Change {
        n124 = event-data() -> ()  [unwired: 1 in, 5 out]
        n125 = call <vilib>:"Open URL in Default Browser (string).vi"("URL"="http://www.scientifica.uk.com/") -> ()  [unwired: 5 in, 2 out]
      }
      event "advanced settings slider tab", "hist/ref slider tab", "PMT slider tab", "laser power slider tab", "XYZ stage settings slider tab": Mouse Enter; "advanced settings slider tab", "hist/ref slider tab", "PMT slider tab", "laser power slider tab", "XYZ stage settings slider tab": Mouse Leave {
        n126 = event-data() -> ("Type"=w164:T16, "CtlRef"=w163:refnum<vi>)  [unwired: 1 in, 1 out]
        n127 = case shown="1, Default" w165 {
          tunnel: [0 w173] -> w166
          tunnel: w164 -> [_ w172]
          tunnel: w164 -> [_ w171]
          tunnel: w163 -> [_ w170]
          tunnel: [w167 w169] -> w162
          tunnel: w161 -> [w167 _]
          frame 0 {
          }
          frame 1, Default {
            n128 = case shown="\"Mouse Leave\", Default" w172 {
              tunnel: [0 150] -> w173
              frame "Mouse Leave", Default {
              }
              frame "Mouse Enter" {
              }
            }
            n129 = Bundle("Type"=w171, "CtlRef"=w170) -> (w169:cluster{"Type":T16, "CtlRef":refnum<vi>})  [unwired: 1 in]
          }
        }
      }
      event "clear prot", "timestamp.prot", "protocol.notes": Value Change {
        n130 = event-data() -> ("CtlRef"=w180:refnum<vi>)  [unwired: 1 in, 4 out]
        n131 = property class="Ctl"(reference=w180) -> ("Label.Text"=w179:string)  [unwired: 1 in, 2 out]
        n132 = case shown="\"clear prot\"" w179 {
          tunnel: "protocol.notes" -> [w181 w183 _]
          tunnel: [w181 w182 ""] -> w177
          frame "Null", Default {
          }
          frame "timestamp.prot" {
            n133 = Get Date/Time In Seconds() -> (seconds since 1Jan1904=w186:timestamp)
            n134 = Format Date/Time String(time format string (%c)="%Y-%m-%d %H:%M:%S%2u", seconds (now)=w186) -> (date/time string=w184:string)  [unwired: 1 in]
            n135 = Concatenate Strings(w183, "\n##################\n" ("string"), w184) -> (w182:string)
          }
          frame "clear prot" {
          }
        }
        n136 = local write "protocol.notes"(w177) -> ()
      }
    }
  }
  n137 = flat-sequence {
    tunnel: w1 -> [_]
    frame #0 {
      w189 = T12."Enabled" ("Disabled")
      # "tab controls"
      n138 = disable-structure shown="Enabled" {
        frame Disabled {
          n139 = call "set and reset slider tabs.vi"("Set(T)/Reset(F)"=TRUE) -> ()  [unwired: 11 in]
        }
        frame Enabled {
        }
      }
      n140 = local write "scan mode main settings"(scan_mode_main_settings_tab."2D frame" ("scan mode main settings")) -> ()
      n141 = Build Array("nomin.x.pixels" ("Variable Name in")) -> (w192:string[])
      n142 = call "GFG refresh all variables.vi"("All Variable Names"=w192) -> ()  [unwired: 11 in]
      n143 = call "init obj.vi"() -> ()  [unwired: 12 in]
      n144 = property on="FOCUS" class="Bool (strict)"("DisabledEnum"=w189) -> ()  [unwired: 2 in, 2 out]
      n145 = property on="Record" class="Bool (strict)"("DisabledEnum"=w189) -> ()  [unwired: 2 in, 2 out]
    }
  }
  n146 = flat-sequence {
    tunnel: w8 -> [w195]
    tunnel: [w195] -> w4
    tunnel: w4 -> [w196]
    frame #0 {
      n147 = call "close modules.vi"("close FP?"=TRUE) -> ()  [unwired: 11 in]
    }
    frame #1 {
      n148 = Not(x=w196) -> (.not. x?=w197:bool)
      n149 = call "ReadGFGandWriteToINI.vi"() -> ("error out"=w198:errorcluster)  [unwired: 11 in]
      n150 = local write "QUIT"(w197) -> ()
      n151 = call "GFG_core.vi"("error in (no error)"=w198, "Action"=enum16{"Init", "Set", "Get"}."Init") -> ()  [unwired: 11 in, 7 out]
    }
    frame #2 {
      n152 = case shown="True" TRUE {
        frame False {
          n153 = Quit LabVIEW(quit? (T)=TRUE) -> ()
        }
        frame True {
          n154 = case shown="False" FALSE {
            frame False {
            }
            frame True {
              n155 = control-ref of="This VI"() -> (w203:refnum<vi>)
              n156 = invoke class="VI" method="FP.Close"(reference=w203) -> ()  [unwired: 2 in, 3 out]
            }
          }
        }
      }
    }
  }
